vi "6134 Counter Config Test.vi"() -> (15 "error out":errorcluster)   [LabVIEW 2015]
uses:
  Type Defs/Counter Params.ctl
  <vilib>/DAQmx/create/channels.llb/DAQmx Create Channel (CO-Pulse Generation-Ticks).vi
  <vilib>/DAQmx/configure/timing.llb/DAQmx Timing (Implicit).vi
  <resource>/objmgr/daqmx.rc
panel:
  in  "source of ticks":tag="OnboardClock"
  in  "counter":tag
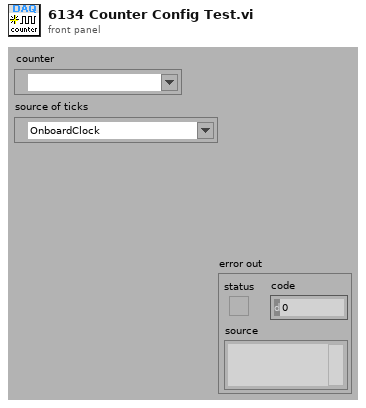
[diagram p1: front panel]
types:
  T1 = typedef "Counter Params.ctl" = cluster{"Counter":tag, "Hi ticks":u32, "Low ticks":u32, "Idle state":i32, "Delay ticks":u32}
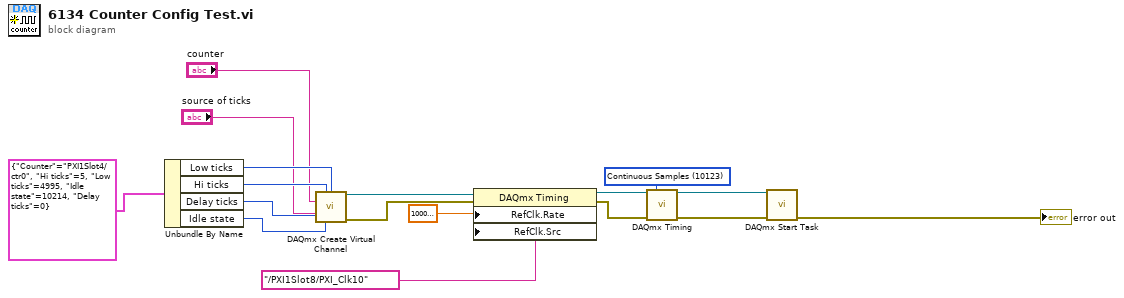
[diagram p0: block diagram]
diagram:
  w17 = 10123 items=["Finite Samples"=10178, "Continuous Samples"=10123] ("sample mode")
  n1 = Unbundle By Name(T1 {"Counter"="PXI1Slot4/ctr0", "Hi ticks"=5, "Low ticks"=4995, "Idle state"=10214, "Delay ticks"=0} ("Counter Parameters")) -> ("Low ticks"=w12:u32, "Hi ticks"=w11:u32, "Delay ticks"=w10:u32, "Idle state"=w9:i32)
  n2 = call-poly <vilib>:"DAQmx Create Virtual Channel.vi"("high ticks"=w11, "low ticks"=w12, "counter"="counter", "source of ticks"="source of ticks", "idle state"=w9, "initial delay"=w10) -> ("task out"=w13:refnum<k21>, "error out"=w14:errorcluster)  [unwired: 8 in]
  n3 = property class="DAQmx Timing"(reference=w13, error in=w14, "RefClk.Rate"=10000000.0, "RefClk.Src"=tag "/PXI1Slot8/PXI_Clk10") -> (reference out=w16:refnum<k21>, error out=w15:errorcluster)
  n4 = call-poly <vilib>:"DAQmx Timing.vi"("task/channels in"=w16, "sample mode"=w17, "error in"=w15) -> ("task out"=w2:refnum<k21>, "error out"=w7:errorcluster)  [unwired: 11 in]
  n5 = call <vilib>:"DAQmx Start Task.vi"("task/channels in"=w2, "error in"=w7) -> ("error out"=→"error out":errorcluster)  [unwired: 12 in, 1 out]
